vi "Data array treatment.vi"(0 "Xdata":sgl[](array[numeric]), 1 "Ydata":sgl[](array[numeric]), 2 "Zero array":sgl[](array[numeric]), 3 "Start \nwavelength":sgl, 4 "End\nwavelength":sgl, 5 "Moving\naverage":i16=1 min=1 step=1, 8 "Transmission":bool, 10 "Crop":bool, 12 "Moving AV":bool, 14 "Normalise":bool) -> (20 "Xdata":dbl[](array[numeric]), 21 "Ydata":dbl[](array[numeric]))   [LabVIEW 2014]
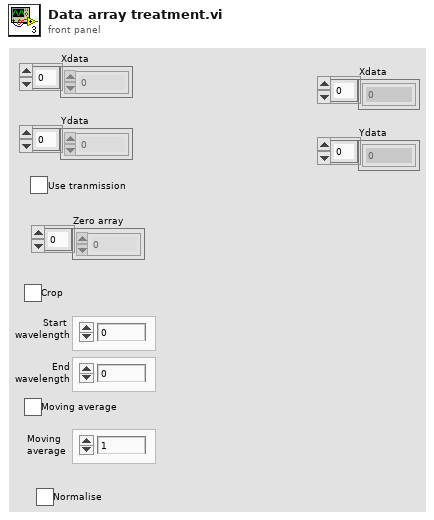
[diagram p1: front panel]
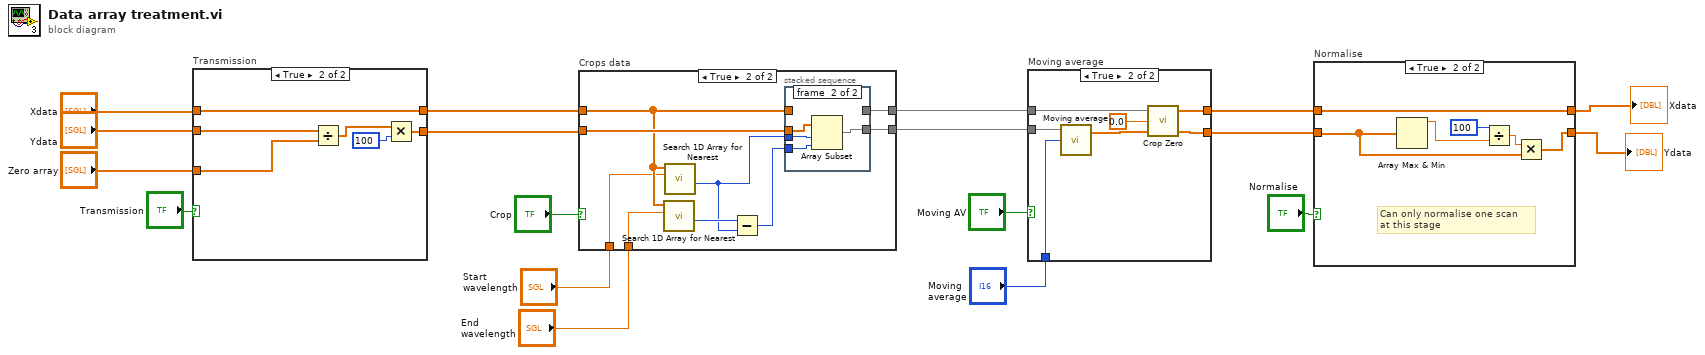
[diagram p0: block diagram]
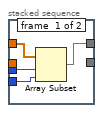
[diagram p6: hidden frame]
diagram:
  n1 = case "Transmission" shown="True" "Transmission" {
    tunnel: "Xdata" -> [w20 w22]
    tunnel: "Ydata" -> [w19 w24]
    tunnel: [w20 w22] -> w9
    tunnel: [w19 w23] -> w10
    tunnel: "Zero array" -> [_ w21]
    frame False {
    }
    frame True {
      n2 = Divide(x=w24, y=w21) -> (x/y=w25:sgl[])
      n3 = Multiply(x=w25, y=100) -> (x*y=w23:sgl[])
    }
  }
  n4 = case "Crops data" shown="True" "Crop" {
    tunnel: w9 -> [w28 w31]
    tunnel: w10 -> [w27 w32]
    tunnel: [w28 w34] -> w6
    tunnel: [w27 w33] -> w7
    tunnel: "Start \nwavelength" -> [_ w30]
    tunnel: "End\nwavelength" -> [_ w29]
    frame False {
    }
    frame True {
      n5 = call "Search 1D Array for Nearest.vi"("desired element"=w29, "1D Array"=w31) -> ("closest index"=w37:i32)  [unwired: 8 in, 1 out]
      n6 = call "Search 1D Array for Nearest.vi"("desired element"=w30, "1D Array"=w31) -> ("closest index"=w36:i32)  [unwired: 8 in, 1 out]
      n7 = Subtract(x=w37, y=w36) -> (x-y=w35:i32)
      n8 = stacked-sequence {
        tunnel: w31 -> [w38 _]
        tunnel: w36 -> [w41 w45]
        tunnel: w35 -> [w40 w44]
        tunnel: w32 -> [_ w42]
        tunnel: [_ w43] -> w33
        tunnel: [w39 _] -> w34
        frame #0 {
          n9 = Array Subset(array=w38, index=w41, length=w40) -> (w39:sgl[])
        }
        frame #1 {
          n10 = Array Subset(array=w42, index=w45, length=w44) -> (w43:sgl[])
        }
      }
    }
  }
  n11 = case "Moving average" shown="True" "Moving AV" {
    tunnel: w6 -> [w47 w50]
    tunnel: w7 -> [w46 w54]
    tunnel: [w47 w52] -> w15
    tunnel: [w46 w51] -> w16
    tunnel: "Moving\naverage" -> [_ w53]
    frame False {
    }
    frame True {
      n12 = call "Moving average.vi"("Width of AV"=w53, "Raw data"=w54) -> ("Data AVs"=w49:dbl[])  [unwired: 1 in, 1 out]
      n13 = call "Crop Zero.vi"("Search data"=w49, "Search value"=0.0, "Paired data"=w50) -> ("Searched data out"=w51:dbl[], "Paired data out"=w52:dbl[])  [unwired: 1 in]
    }
  }
  n14 = case "Normalise" shown="True" "Normalise" {
    tunnel: w15 -> [w55 w58]
    tunnel: w16 -> [w56 w59]
    tunnel: [w55 w58] -> w18
    tunnel: [w56 w57] -> w17
    frame False {
    }
    frame True {
      # "Can only normalise one scan\nat this stage"
      n15 = Array Max & Min(array=w59) -> (max value=w62:dbl)  [unwired: 3 out]
      n16 = Divide(x=100, y=w62) -> (x/y=w60:dbl)
      n17 = Multiply(x=w60, y=w59) -> (x*y=w57:dbl[])
    }
  }
  "Xdata" <- w18
  "Ydata" <- w17
